vi "Sandwich.vi"(0 "Pince control teleop":bool) -> ()   [LabVIEW 2017]
uses:
  <vilib>/Rock Robotics/WPI/Solenoid/WPI_SolenoidValue.ctl
  Robot Global Data.vi
  <vilib>/Rock Robotics/WPI/Solenoid/WPI_SolenoidSetEnum.vi
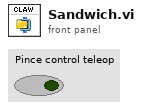
[diagram p1: front panel]
types:
  T1 = typedef "WPI_SolenoidValue.ctl" = enum16{"Off", "On", "Forward", "Reverse"}
  T2 = typedef "WPI_SolenoidDevRef.ctl" = cluster{"DevStatus":errorcluster, "Pneumatics Control Module":u8, "Forward Solenoid Channel":T3, "Reverse Solenoid Channel":T3}
  T3 = typedef "WPI_SolenoidChannel.ctl" = enum8{"Solenoid 0", "Solenoid 1", "Solenoid 2", "Solenoid 3", "Solenoid 4", "Solenoid 5", "Solenoid 6", "Solenoid 7", "Invalid"}
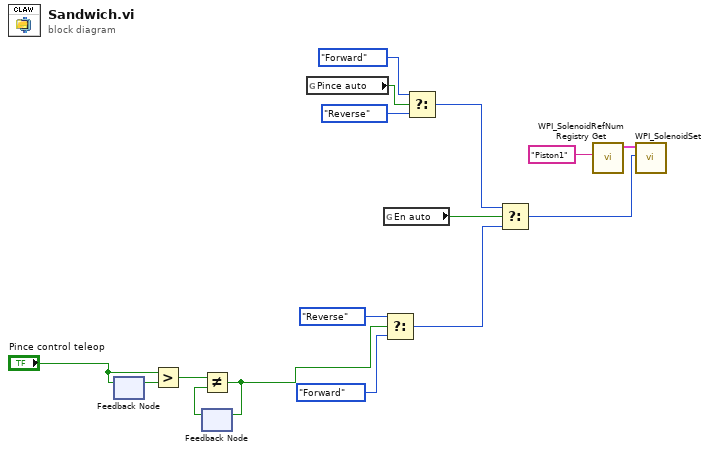
[diagram p0: block diagram]
diagram:
  n1 = feedback #1() -> (w5:bool)  [unwired: 1 in]
  n2 = feedback-in #1("Pince control teleop") -> ()
  n3 = Greater?(x="Pince control teleop", y=w5) -> (0:w4:bool)
  n4 = feedback #2() -> (w3:bool)  [unwired: 1 in]
  n5 = Not Equal?(x=w4, y=w3) -> (x != y?=w2:bool)
  n6 = feedback-in #2(w2) -> ()
  n7 = global read "Robot Global Data.vi" "Pince auto"() -> (w7:bool)
  n8 = global read "Robot Global Data.vi" "En auto"() -> (w12:bool)
  n9 = Select(t=WPI_SolenoidValue."Reverse" ("Value"), s=w2, f=WPI_SolenoidValue."Forward" ("Value")) -> (s? t:f=w11:T1)
  n10 = Select(t=WPI_SolenoidValue."Forward" ("Value"), s=w7, f=WPI_SolenoidValue."Reverse" ("Value")) -> (s? t:f=w8:T1)
  n11 = Select(t=w8, s=w12, f=w11) -> (s? t:f=w6:T1)
  n12 = call <vilib>:"WPI_SolenoidRefNum Registry Get.vi"("refnum name"="Piston1") -> ("SolenoidDevRef"=w14:T2)  [unwired: 9 in, 1 out]
  n13 = call-poly <vilib>:"WPI_SolenoidSet.vi"("Value"=w6, "SolenoidDevRef"=w14) -> ()  [unwired: 8 in, 2 out]
